vi "Sample1.vi"   [LabVIEW 2014]
types:
  T1 = enum16{"Add User Event Ref", "Get User Event Ref", "Delete User Event Ref", "Get All User Event Refs", "Delete All User Event Refs"}
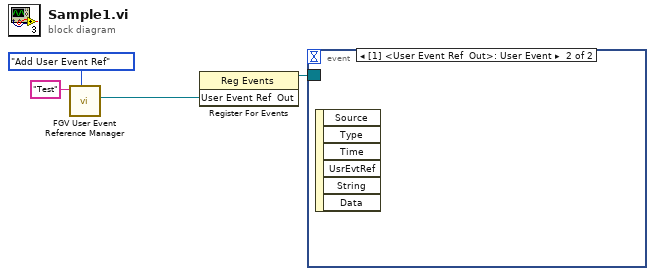
[diagram p0: block diagram]
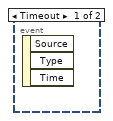
[diagram p2: hidden frame]
diagram:
  n1 = call "FGV User Event Reference Manager.vi"("Method (Get User Event Ref)"=T1."Add User Event Ref", "User Event Name"="Test") -> ("User Event Ref  Out"=w1:refnum<user-event>)  [unwired: 6 in, 3 out]
  n2 = register-events(w1) -> (reference out=w2:refnum<event-registration>)  [unwired: 2 in, 1 out]
  n3 = event shown="[1] <User Event Ref  Out>: User Event" {
    selector: w2 -> [_ _]
    dyn-events: _ -> [_ _]
    timeout: _ -> [_ _]
    event Timeout {
      n4 = event-data() -> ()  [unwired: 1 in, 3 out]
    }
    event User Event {
      n5 = event-data() -> ()  [unwired: 1 in, 6 out]
    }
  }
